vi "Simple 2-color Interpolation Palette.vi"(8 "Error In":errorcluster, 10 "Scale.Low Color":u32, 11 "Scale.High Color":u32) -> (0 "Error Out":errorcluster, 3 "Scale.MarkerVals[0-255]":cluster{i32, "Color":u32}[](array[cluster]))   [LabVIEW 2021, in "Palette.lvlib"]
uses:
  Palette.lvlib
panel:
  out "Color Ramp":dbl(ramp)
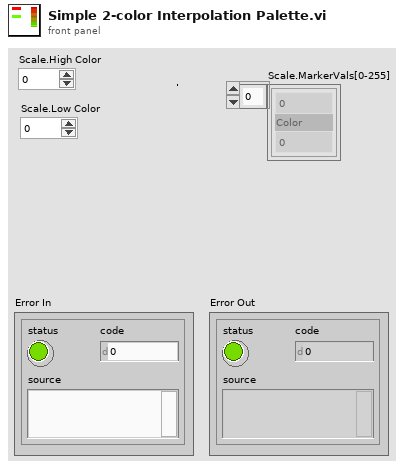
[diagram p1: front panel]
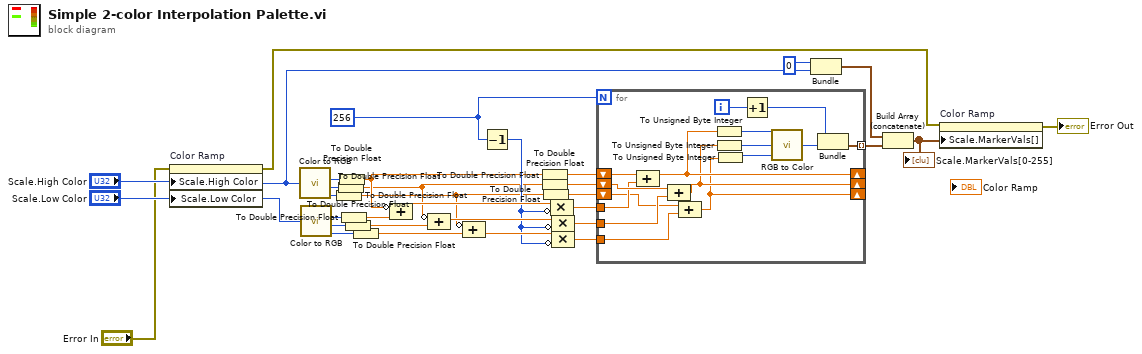
[diagram p0: block diagram]
diagram:
  w26 = 256
  n1 = property on="Color Ramp" class="ColRmp (strict)"(error in="Error In", "Scale.High Color"="Scale.High Color", "Scale.Low Color"="Scale.Low Color") -> (error out=w2:errorcluster)  [unwired: 1 in, 1 out]
  n2 = call <vilib>:"Color to RGB.vi"("Color"="Scale.High Color") -> ("R"=w12:u8, "G"=w32:u8, "B"=w28:u8)  [unwired: 1 out]
  n3 = call <vilib>:"Color to RGB.vi"("Color"="Scale.Low Color") -> ("R"=w31:u8, "G"=w30:u8, "B"=w29:u8)  [unwired: 1 out]
  n4 = To Double Precision Float(number=w28) -> (double precision float=w9:dbl)
  n5 = To Double Precision Float(number=w32) -> (double precision float=w10:dbl)
  n6 = To Double Precision Float(number=w12) -> (double precision float=w11:dbl)
  n7 = To Double Precision Float(number=w31) -> (double precision float=w8:dbl)
  n8 = To Double Precision Float(number=w30) -> (double precision float=w7:dbl)
  n9 = To Double Precision Float(number=w29) -> (double precision float=w6:dbl)
  n10 = Compound Arithmetic op=ADD(invert w11, w8) -> (w21:dbl)
  n11 = Compound Arithmetic op=ADD(invert w10, w7) -> (w20:dbl)
  n12 = Compound Arithmetic op=ADD(invert w9, w6) -> (w27:dbl)
  n13 = Decrement(x=w26) -> (x-1=w19:i32)
  n14 = To Double Precision Float(number=w11) -> (double precision float=w24:dbl)
  n15 = To Double Precision Float(number=w10) -> (double precision float=w23:dbl)
  n16 = To Double Precision Float(number=w9) -> (double precision float=w22:dbl)
  n17 = Compound Arithmetic op=MULTIPLY(w21, invert w19) -> (w18:dbl)
  n18 = Compound Arithmetic op=MULTIPLY(w20, invert w19) -> (w17:dbl)
  n19 = Compound Arithmetic op=MULTIPLY(w27, invert w19) -> (w25:dbl)
  n20 = for {
    N: w26 -> [_]
    shift-right: [w42] -> _
    shift-left: w24 -> [w43]
    shift-right: [w41] -> _
    shift-left: w23 -> [w48]
    shift-right: [w40] -> _
    shift-left: w22 -> [w44]
    tunnel: w25 -> [w45]
    tunnel: w18 -> [w47]
    tunnel: w17 -> [w46]
    tunnel: [w35] -> w16 mode=indexing
    i -> [w34]
    n21 = Compound Arithmetic op=ADD(w43, w47) -> (w42:dbl)
    n22 = Compound Arithmetic op=ADD(w48, w46) -> (w41:dbl)
    n23 = Compound Arithmetic op=ADD(w44, w45) -> (w40:dbl)
    n24 = To Unsigned Byte Integer(number=w42) -> (unsigned 8bit integer=w39:u8)
    n25 = To Unsigned Byte Integer(number=w41) -> (unsigned 8bit integer=w38:u8)
    n26 = To Unsigned Byte Integer(number=w40) -> (unsigned 8bit integer=w37:u8)
    n27 = Increment(x=w34) -> (x+1=w33:i32)
    n28 = call <vilib>:"RGB to Color.vi"("B"=w37, "G"=w38, "R"=w39) -> ("Color"=w36:u32)
    n29 = Bundle(w33, "Color"=w36) -> (w35:cluster{i32, "Color":u32})  [unwired: 1 in]
  }
  n30 = Bundle(0, "Scale.High Color"="Scale.High Color") -> (w14:cluster{i32, "Scale.High Color":u32})  [unwired: 1 in]
  n31 = Build Array (concatenate)(w14, w16) -> (w13:cluster{i32, "Color":u32}[])
  "Scale.MarkerVals[0-255]" <- w13
  n32 = property on="Color Ramp" class="ColRmp (strict)"(error in=w2, "Scale.MarkerVals[]"=w13) -> (error out=→"Error Out":errorcluster)  [unwired: 1 in, 1 out]
